vi "Express DAQ.vi"() -> ()   [LabVIEW 2025]
panel:
  in  "Stop":bool
  in  "Write":bool
  out "Read":bool
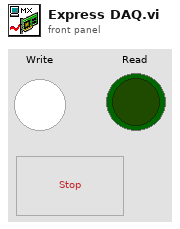
[diagram p1: front panel]
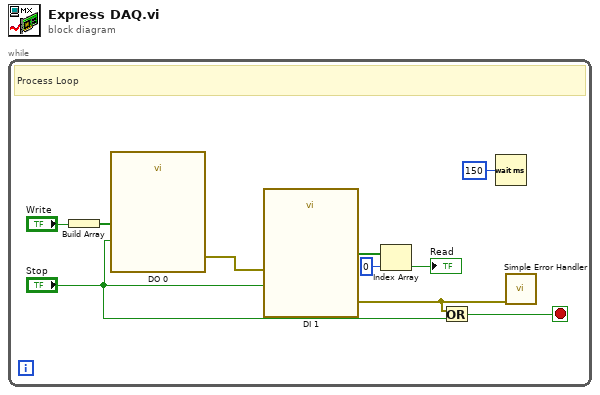
[diagram p0: block diagram]
diagram:
  n1 = while {
    stop <- w9 stop-if-true
    # "Process Loop"
    n2 = Build Array("Write") -> (w7:bool[])
    n3 = call "DO 0"("data"=w7, "stop (T)"="Stop") -> ("error out"=w3:errorcluster)  [unwired: 16 in, 1 out]
    n4 = call "DI 1"("error in"=w3, "stop (T)"="Stop") -> ("data"=w6:bool[], "error out"=w1:errorcluster)  [unwired: 15 in, 1 out]
    n5 = Index Array(array=w6, index=0) -> (element=→"Read":bool)
    n6 = Or(x=w1, y="Stop") -> (x .or. y?=w9:bool)
    n7 = Wait (ms)(milliseconds to wait=u32 150) -> ()  [unwired: 1 out]
    n8 = call <vilib>:"Simple Error Handler.vi"("error in (no error)"=w1) -> ()  [unwired: 4 in, 5 out]
  }
